vi "LOGIC_writeSubstracted.vi"(0 "total pixels":u32, 1 "log file":path, 2 "write":bool, 5 "bpp":i16, 7 "subs buf":u64, 9 "name":string, 11 "error in (no error)":errorcluster) -> (15 "error out":errorcluster)   [LabVIEW 2016]
uses:
  Common/public/vis/CMN_FVAR_action.ctl
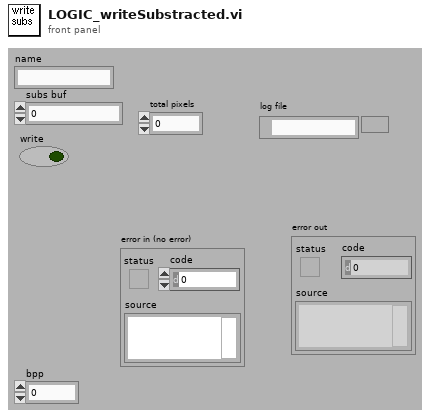
[diagram p1: front panel]
types:
  T1 = typedef "CMN_FVAR_action.ctl" = enum16{"read", "write"}
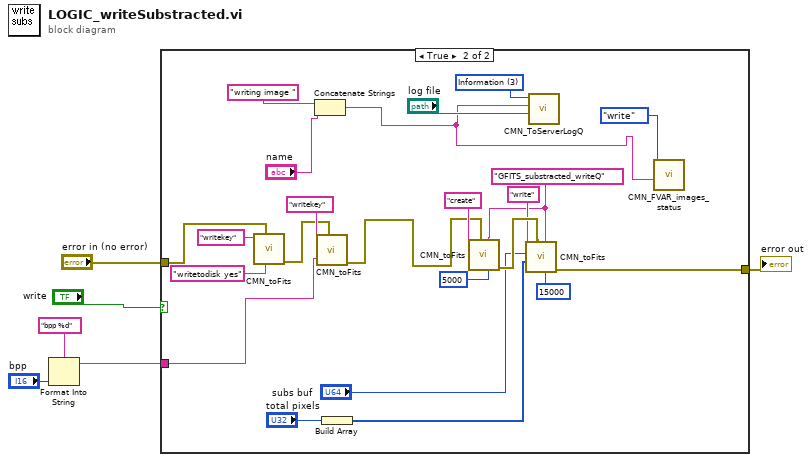
[diagram p0: block diagram]
diagram:
  n1 = Format Into String(format string="bpp %d" ("key"), "bpp") -> (resulting string=w1:string)  [unwired: 2 in, 1 out]
  n2 = case shown="True" "write" {
    tunnel: "error in (no error)" -> [w7 w22]
    tunnel: [w7 w21] -> w5
    tunnel: w1 -> [_ w12]
    frame False {
    }
    frame True {
      w17 = u16 3 items=["command", "imediateReply", "Callback Reply", "Information"] ("type")
      w13 = "GFITS_substracted_writeQ" ("response Q")
      n3 = call "CMN_toFits.vi"("key"="writetodisk yes", "error in (no error)"=w22, "command"="writekey") -> ("error out"=w25:errorcluster)  [unwired: 5 in, 3 out]
      n4 = Concatenate Strings("writing image ", "name") -> (w9:string)
      n5 = call "CMN_toFits.vi"("key"=w12, "error in (no error)"=w25, "command"="writekey") -> ("error out"=w11:errorcluster)  [unwired: 5 in, 3 out]
      n6 = Build Array("total pixels") -> (w20:u32[])
      n7 = call "CMN_toFits.vi"("ms timeout (-1)"=5000, "response Q"=w13, "error in (no error)"=w11, "command"="create") -> ("error out"=w28:errorcluster)  [unwired: 4 in, 3 out]
      n8 = call "CMN_toFits.vi"("ms timeout (-1)"=15000, "response Q"=w13, "error in (no error)"=w28, "eleRead"=w20, "location"="subs buf", "command"="write") -> ("error out"=w21:errorcluster)  [unwired: 2 in, 3 out]
      n9 = call "CMN_ToServerLogQ.vi"("file"="log file", "string"=w9, "type"=w17) -> ()  [unwired: 3 in, 5 out]
      n10 = call "CMN_FVAR_images_status.vi"("value in"=w9, "action"=CMN_FVAR_action."write") -> ()  [unwired: 9 out]
    }
  }
  "error out" <- w5
